vi "Swerve Wheel.vi"(1 "Wheel":T2(ring)=enum."Front Right", 2 "Inputs":dbl[](array[numeric])=[0.0, -0.10193669212665253, -0.14931439584198622, 0.0, 0.0, 10.75, 15.027058927148719, 10.5], 3 "br offset":dbl(knob)=-6.7034593303000065 scale=-180.0..180.0, 4 "bl offset":dbl(knob)=27.320075486284452 scale=-180.0..180.0, 5 "fr offset":dbl(knob)=31.44769799349993 scale=-180.0..180.0, 6 "fl offset":dbl(knob)=31.73032709235852 scale=-180.0..180.0) -> (0 "Speed":dbl=0.1807923615847232)   [LabVIEW 2017]
uses:
  <vilib>/Rock Robotics/WPI/ThirdParty/Phoenix-LabVIEW/Motor Controller/Controls/CTRE_Phoenix_MotorControl_ControlMode.ctl
  <vilib>/Rock Robotics/Network Tables/NT Write Number.vi
  <vilib>/addons/control/pid/pid.llb/PID (DBL).vi
  <vilib>/Rock Robotics/WPI/ThirdParty/Phoenix-LabVIEW/Motor Controller/Get/CTRE_Phoenix_MotorController_GetAnalogData.vi
  <vilib>/addons/control/pid/NI_PID_pid.lvlib
panel:
  out "angle":dbl
  in  "PID gains":T1={"proportional gain (Kc)"=0.008, "integral time (Ti, min)"=0.0, "derivative time (Td, min)"=0.1}
  # "Practice Robot Offsets (3-27-17)\n\nFL:  33\nFR: 32\nBL: 30\nBR:  -178"
  # "Gamer Bot Offsets (3/29/17)\n\nFL: -.7\nFR: -165.5\nBL: 98.2\nBR: -66.7"
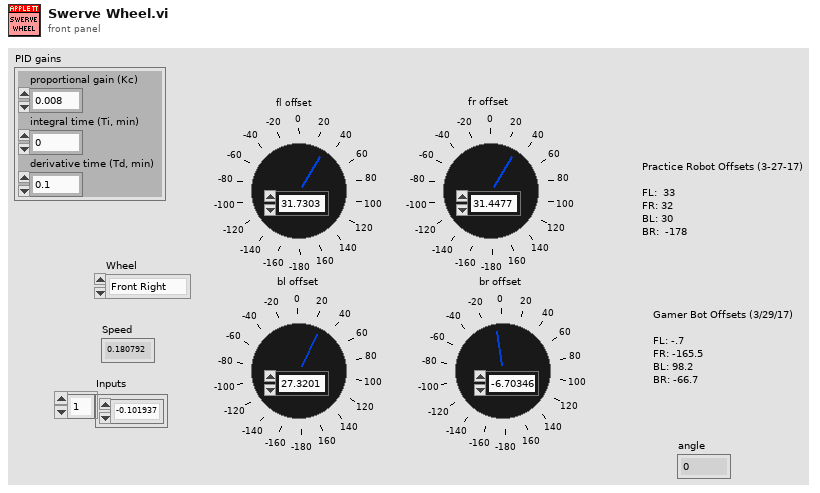
[diagram p1: front panel]
types:
  T1 = cluster{"proportional gain (Kc)":dbl, "integral time (Ti, min)":dbl, "derivative time (Td, min)":dbl}
  T2 = enum16{"Back Left", "Back Right", "Front Left", "Front Right"}
  T3 = typedef "CTRE_Phoenix_MotorControl_ControlMode.ctl" = u16
  T4 = enum16{"Z", "Y", "X", "Rot. Point X", "Rot. Point Y", "Width/2", "Max", "Length/2"}
  T5 = enum16{"Z Axis", "Y", "X", "Rot. Point X", "Rot. Point Y", "Width/2", "Max", "Length/2"}
  T6 = typedef "WPI_MotorControlDeviceRef.ctl" = cluster{"DeviceStatus":errorcluster, "Type":T7, "PWM":cluster{"PWM Channel":T8, "DeadBand":T9}, "CAN":cluster{"Device Number":u8, "SetOutput VI Ref":variant, "GetOutput VI Ref":variant, "Enable VI Ref":variant, "Disable VI Ref":variant, "Data":variant}, "Invert":bool, "DIO PWM":cluster{"PWM \"Enable\" Channel":T8, "DIOChannel":T10, "PWM Rate":dbl}}
  T7 = typedef "WPI_MotorControlType.ctl" = enum16{"PWM", "CAN", "DIO PWM"}
  T8 = typedef "FPGA_DIOPWMChannel.ctl" = enum8{"PWM 0", "PWM 1", "PWM 2", "PWM 3", "PWM 4", "PWM 5", "PWM 6", "PWM 7", "PWM 8", "PWM 9", "PWM MXP 0", "PWM MXP 1", "PWM MXP 2", "PWM MXP 3", "PWM MXP 4", "PWM MXP 5", "PWM MXP 6", "PWM MXP 7", "PWM MXP 8", "PWM MXP 9", "Invalid"}
  T9 = typedef "WPI_PWMDeadband.ctl" = cluster{"Name":string, "maxPositivePwm":i32, "minPositivePwm":i32, "centerPwm":i32, "maxNegativePwm":i32, "minNegativePwm":i32, "angularRange":u16}
  T10 = typedef "FPGA_DIOChannel.ctl" = enum8{"DIO 0", "DIO 1", "DIO 2", "DIO 3", "DIO 4", "DIO 5", "DIO 6", "DIO 7", "DIO 8", "DIO 9", "DIO MXP 0", "DIO MXP 1", "DIO MXP 2", "DIO MXP 3", "DIO MXP 4", "DIO MXP 5", "DIO MXP 6", "DIO MXP 7", "DIO MXP 8", "DIO MXP 9", "DIO MXP 10", "DIO MXP 11", "DIO MXP 12", "DIO MXP 13", "DIO MXP 14", "DIO MXP 15", "SPI Port CS1", "SPI Port CS2", "SPI Port CS3", "SPI Port MISO", "SPI Port MOSI", "Invalid"}
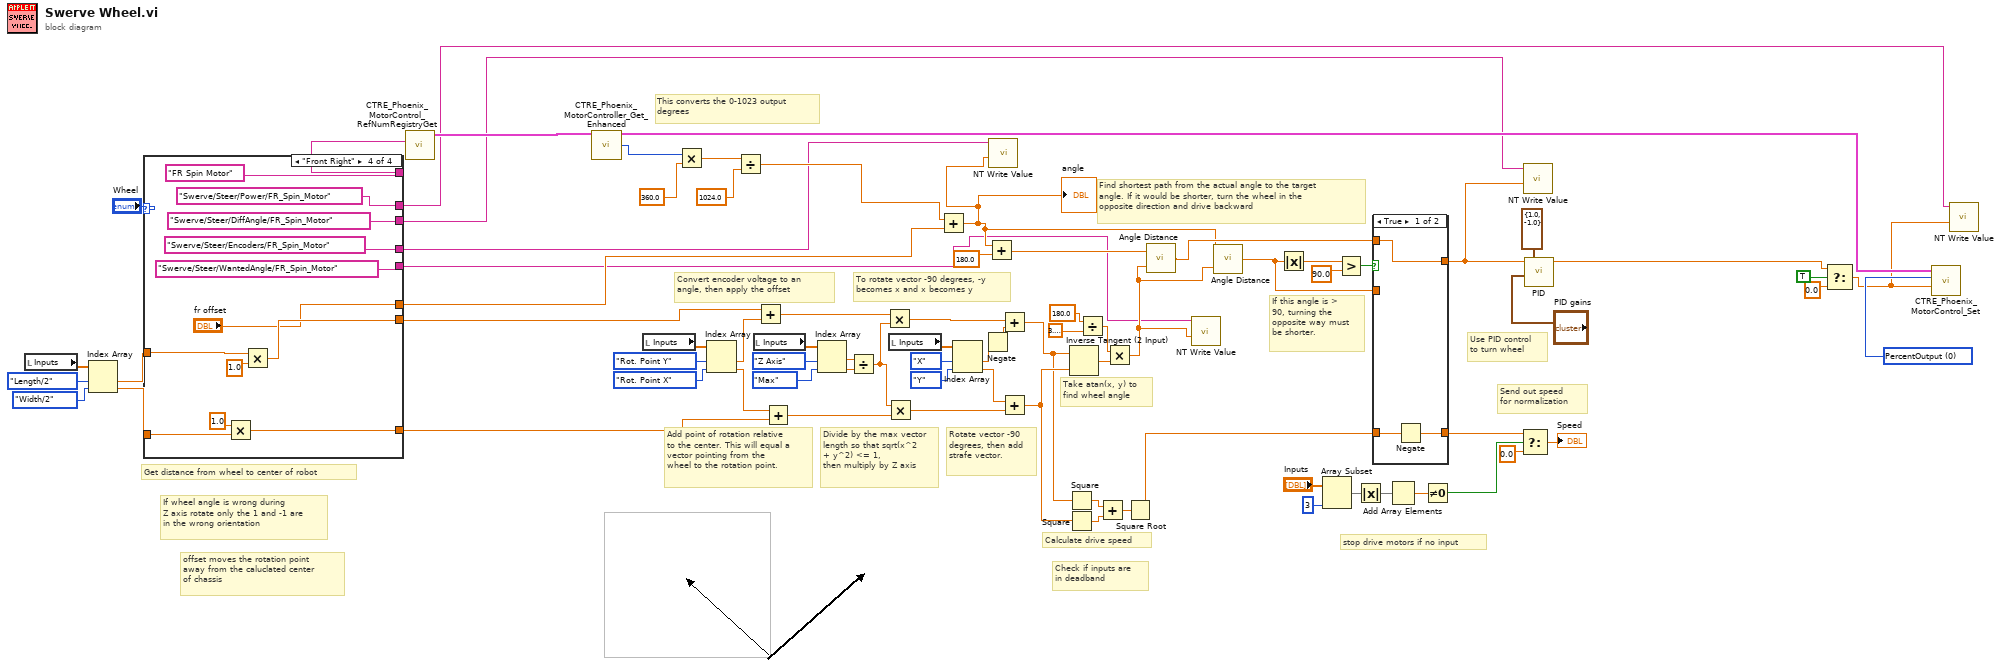
[diagram p0: block diagram]
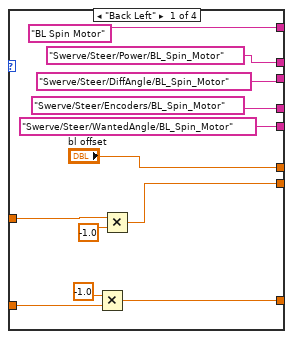
[diagram p3: hidden frame]
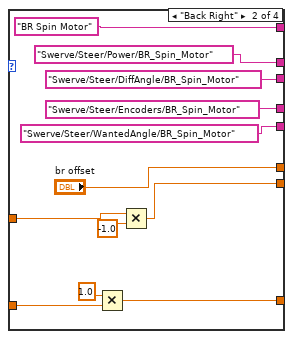
[diagram p4: hidden frame]
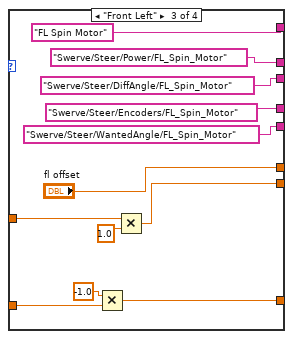
[diagram p5: hidden frame]
diagram:
  w12 = T3 0 items=["PercentOutput"=0, "Position"=1, "Velocity"=2, "Current"=3, "Follower"=5, "MotionProfile"=6, "MotionMagic"=7, "MotionMagicArc"=8, "MotionProfileArc"=10, "Disabled"=15] ("Control Mode")
  # "stop drive motors if no input"
  # "This converts the 0-1023 output \ndegrees"
  # "offset moves the rotation point\naway from the caluclated center\nof chassis"
  # "If wheel angle is wrong during\nZ axis rotate only the 1 and -1 are\nin the wrong orientation"
  # "To rotate vector -90 degrees, -y becomes x and x becomes y"
  # "Divide by the max vector length so that sqrt(x^2 + y^2) <= 1,\nthen multiply by Z axis"
  # "Add point of rotation relative to the center. This will equal a vector pointing from the\nwheel to the rotation point."
  # "Send out speed\nfor normalization"
  # "Check if inputs are\nin deadband"
  # "Convert encoder voltage to an angle, then apply the offset"
  # "If this angle is > 90, turning the opposite way must be shorter."
  # "Use PID control\nto turn wheel"
  # "Find shortest path from the actual angle to the target angle. If it would be shorter, turn the wheel in the opposite direction and drive backward"
  # "Take atan(x, y) to find wheel angle"
  # "Calculate drive speed"
  # "Rotate vector -90 degrees, then add strafe vector."
  # "Get distance from wheel to center of robot"
  n1 = local read "Inputs"() -> (w32:dbl[])
  n2 = Index Array(array=w32, index #1=T4."Length/2", index #2=T4."Width/2") -> (element #1=w30:dbl, element #2=w29:dbl)
  n3 = case shown="\"Front Right\"" "Wheel" {
    tunnel: ["BL Spin Motor" "BR Spin Motor" "FL Spin Motor" "FR Spin Motor"] -> w65
    tunnel: ["bl offset" "br offset" "fl offset" "fr offset"] -> w22
    tunnel: w30 -> [w88 w100 w112 w124]
    tunnel: w29 -> [w86 w98 w111 w122]
    tunnel: [w85 w97 w110 w121] -> w54
    tunnel: [w84 w96 w109 w120] -> w50
    tunnel: ["Swerve/Steer/Encoders/BL_Spin_Motor" "Swerve/Steer/Encoders/BR_Spin_Motor" "Swerve/Steer/Encoders/FL_Spin_Motor" "Swerve/Steer/Encoders/FR_Spin_Motor"] -> w8
    tunnel: ["Swerve/Steer/WantedAngle/BL_Spin_Motor" "Swerve/Steer/WantedAngle/BR_Spin_Motor" "Swerve/Steer/WantedAngle/FL_Spin_Motor" "Swerve/Steer/WantedAngle/FR_Spin_Motor"] -> w6
    tunnel: ["Swerve/Steer/DiffAngle/BL_Spin_Motor" "Swerve/Steer/DiffAngle/BR_Spin_Motor" "Swerve/Steer/DiffAngle/FL_Spin_Motor" "Swerve/Steer/DiffAngle/FR_Spin_Motor"] -> w3
    tunnel: ["Swerve/Steer/Power/BL_Spin_Motor" "Swerve/Steer/Power/BR_Spin_Motor" "Swerve/Steer/Power/FL_Spin_Motor" "Swerve/Steer/Power/FR_Spin_Motor"] -> w1
    frame "Back Left" {
      n4 = Multiply(x=-1.0 ("y"), y=w86) -> (x*y=w84:dbl)
      n5 = Multiply(x=w88, y=-1.0) -> (x*y=w85:dbl)
    }
    frame "Back Right" {
      n6 = Multiply(x=1.0 ("y"), y=w98) -> (x*y=w96:dbl)
      n7 = Multiply(x=w100, y=-1.0) -> (x*y=w97:dbl)
    }
    frame "Front Left" {
      n8 = Multiply(x=-1.0 ("y"), y=w111) -> (x*y=w109:dbl)
      n9 = Multiply(x=w112, y=1.0) -> (x*y=w110:dbl)
    }
    frame "Front Right" {
      n10 = Multiply(x=1.0 ("y"), y=w122) -> (x*y=w120:dbl)
      n11 = Multiply(x=w124, y=1.0) -> (x*y=w121:dbl)
    }
  }
  n12 = call <vilib>:"CTRE_Phoenix_MotorControl_RefNumRegistryGet.vi"("refnum name"=w65) -> ("PhoenixMotorControlDevRef"=w21:T6)  [unwired: 9 in, 1 out]
  n13 = call-poly <vilib>:"CTRE_Phoenix_MotorController_Get_Enhanced.vi"("PhoenixMotorControlDevRef"=w21) -> ("PhoenixMotorControlDevRef"=w20:T6, "AnalogInRaw"=w16:i32)  [unwired: 10 in, 3 out]
  n14 = local read "Inputs"() -> (w52:dbl[])
  n15 = Multiply(x=w16, y=360.0) -> (x*y=w14:dbl)
  n16 = Index Array(array=w52, index #1=T4."Rot. Point Y", index #2=T4."Rot. Point X") -> (element #1=w48:dbl, element #2=w49:dbl)
  n17 = Divide(x=w14, y=1024.0) -> (x/y=w11:dbl)
  n18 = local read "Inputs"() -> (w46:dbl[])
  n19 = Add(x=w54, y=w48) -> (x+y=w28:dbl)
  n20 = Add(x=w49, y=w50) -> (x+y=w42:dbl)
  n21 = Index Array(array=w46, index #1=T5."Z Axis", index #2=T4."Max") -> (element #1=w43:dbl, element #2=w44:dbl)
  n22 = Divide(x=w43, y=w44) -> (x/y=w10:dbl)
  n23 = Multiply(x=w28, y=w10) -> (x*y=w25:dbl)
  n24 = Multiply(x=w10, y=w42) -> (x*y=w37:dbl)
  n25 = local read "Inputs"() -> (w40:dbl[])
  n26 = Add(x=w11, y=w22) -> (x+y=w9:dbl)
  "angle" <- w9
  n27 = Index Array(array=w40, index #1=T4."X", index #2=T4."Y") -> (element #1=w23:dbl, element #2=w36:dbl)
  n28 = Negate(x=w23) -> (-x=w24:dbl)
  n29 = Add(x=w9, y=180.0 ("f")) -> (x+y=w18:dbl)
  n30 = call-poly <vilib>:"NT Write Value.vi"("Numeric"=w9, "Name"=w8) -> ()  [unwired: 9 in, 1 out]
  n31 = Add(x=w25, y=w24) -> (x+y=w34:dbl)
  n32 = Add(x=w36, y=w37) -> (x+y=w35:dbl)
  n33 = Square(x=w34) -> (x^2=w38:dbl)
  n34 = Square(x=w35) -> (x^2=w74:dbl)
  n35 = Inverse Tangent (2 Input)(1:w35, 2:w34) -> (0:w75:dbl)
  n36 = Divide(x=180.0 ("y"), y=3.141592653589793) -> (x/y=w72:dbl)
  n37 = Add(x=w38, y=w74) -> (x+y=w73:dbl)
  n38 = Multiply(x=w72, y=w75) -> (x*y=w7:dbl)
  n39 = Square Root(x=w73) -> (sqrt(x)=w66:dbl)
  n40 = call "Angle Distance.vi"("target angle"=w7, "current angle"=w18) -> ("distance"=w17:dbl)
  n41 = call-poly <vilib>:"NT Write Value.vi"("Numeric"=w7, "Name"=w6) -> ()  [unwired: 9 in, 1 out]
  n42 = call "Angle Distance.vi"("target angle"=w7, "current angle"=w9) -> ("distance"=w19:dbl)
  n43 = Absolute Value(x=w19) -> (abs(x)=w67:dbl)
  n44 = Array Subset(array="Inputs", length=3) -> (w61:dbl[])  [unwired: 1 in]
  n45 = Greater?(x=w67, y=90.0) -> (0:w57:bool)
  n46 = Absolute Value(x=w61) -> (abs(x)=w55:dbl[])
  n47 = case shown="True" w57 {
    tunnel: w17 -> [w127 _]
    tunnel: w19 -> [_ w131]
    tunnel: [w128 w130] -> w60
    tunnel: w66 -> [w129 w130]
    tunnel: [w127 w131] -> w4
    frame True {
      n48 = Negate(x=w129) -> (-x=w128:dbl)
    }
    frame False {
    }
  }
  n49 = Add Array Elements(numeric array=w55) -> (sum=w76:dbl)
  n50 = Not Equal To 0?(x=w76) -> (x != 0?=w56:bool)
  n51 = Select(t=w60, s=w56, f=0.0) -> (s? t:f=→"Speed":dbl)
  n52 = call-poly <vilib>:"NT Write Value.vi"("Numeric"=w4, "Name"=w3) -> ()  [unwired: 9 in, 1 out]
  n53 = call-poly <vilib>:"PID.vi"("output range"=cluster{"output high":dbl, "output low":dbl} {"output high"=1.0, "output low"=-1.0}, "PID gains"="PID gains", "setpoint"=w4) -> ("output"=w26:dbl)  [unwired: 7 in, 1 out]
  n54 = Select(t=w26, s=TRUE, f=0.0) -> (s? t:f=w2:dbl)
  n55 = call <vilib>:"CTRE_Phoenix_MotorControl_Set.vi"("Output"=w2, "Control Mode"=w12, "PhoenixMotorControlDevRef"=w20) -> ()  [unwired: 7 in, 2 out]
  n56 = call-poly <vilib>:"NT Write Value.vi"("Numeric"=w2, "Name"=w1) -> ()  [unwired: 9 in, 1 out]
